vi "Speed Estimation (N Motors).vi"(0 "waveforms":waveform(dbl)[](array[waveform]), 1 "fundamental frequency [Hz]":dbl=50.0, 2 "reset? (F)":bool, 7 "speed estimation settings":cluster{"% overlap":dbl, "algorithm":T2}={"% overlap"=0.0, "algorithm"=enum."3-phase signals"}, 11 "error in (no error)":errorcluster, 12 "nameplate information":T1, 13 "window length (60 s)":dbl=60.0) -> (3 "new data available?":bool, 4 "speed [RPM]":dbl[](array[numeric]), 6 "slip":dbl[](array[numeric]), 15 "error out":errorcluster)   [LabVIEW 2014, in "NI_EP_Motor Monitoring.lvlib"]
doc: "Calculates the motor speed. You must manually select the polymorphic instance you want to use."
uses:
  <vilib>/addons/Electrical Power/Motor Monitoring/NI_EP_Motor Monitoring.lvlib
  <vilib>/addons/Electrical Power/Motor Monitoring/subVIs/ep_Demodulation Algorithm.ctl
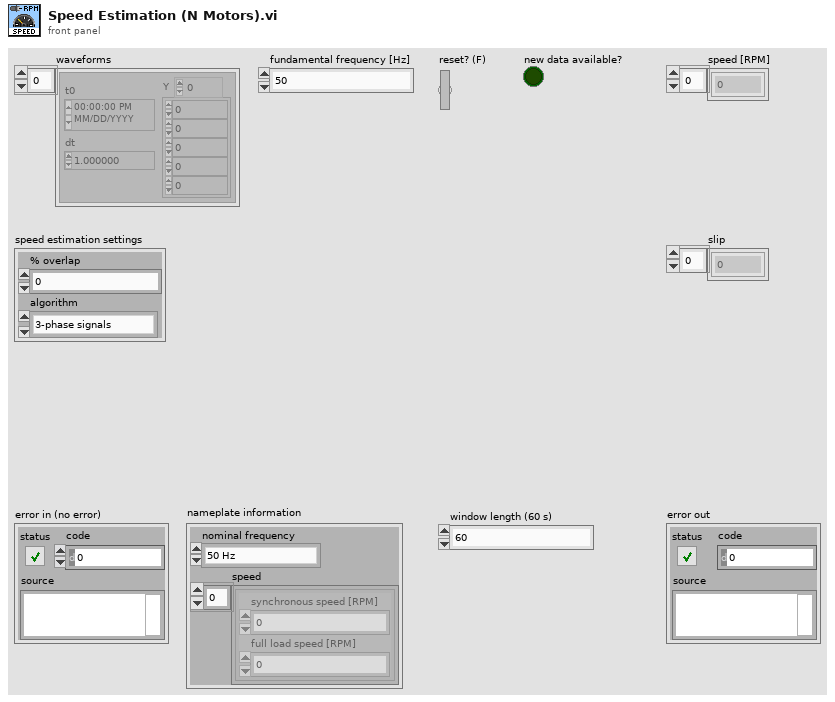
[diagram p1: front panel]
types:
  T1 = cluster{"nominal frequency":enum16{"50 Hz", "60 Hz"}, "speed":cluster{"synchronous speed [RPM]":dbl, "full load speed [RPM]":dbl}[]}
  T2 = typedef "NI_EP_Motor Monitoring.lvlib/ep_Demodulation Algorithm.ctl" = enum16{"1-phase signal", "3-phase signals"}
  T3 = cluster{"block size":i32, "window length [s]":dbl, "dt":dbl}
  T4 = cluster{"synchronous speed [RPM]":dbl, "full load speed [RPM]":dbl}[]
  T5 = typedef "NI_EP_Motor Monitoring.lvlib/ep_Initial Conditions for Speed Estimation.ctl" = cluster{"SVAF state":cluster{"space vector amplitude":dbl, "hilbert state":cluster{"delay conditions":dbl[], "filter conditions":dbl[]}}, "zoom FFT state":cluster{"phase state":dbl, "zoom FFT state":cluster{"zoom settings state":cluster{"zoom":i32, "stop band attenuation":enum16{"84 dB", "96 dB", "120 dB"}, "alias protect in final transition":bool, "oversampling ratio":dbl}, "SML Decimation Filter (complex input) state":cluster{"decimation settings state":cluster{"M":i32, "stop band attenuation":enum16{"84 dB", "96 dB", "120 dB"}, "alias protect in transition band":bool, "oversampling ratio":dbl}, "counter for garbage samples state":i32, "sml_Parameter Setting for Zoom Factor state":cluster{"filter length * interpolation state":i32, "interpolation state":i32, "comb filter order state":i32, "CFIR par state":cluster{"h":dbl[], "M":i32, "N":i32}, "LFIR par state":cluster{"h":dbl[], "M":i32, "N":i32}, "CIC Stages state":i32}, "aal_CIC (complex input) state":cluster{"aal_cascaded moving average (complex input) state":cluster{"states":cdb[], "circular buffers state":cdb[][], "circular buffer counter state":i32}, "aal_moving average with decimation by order (complex input) state":cluster{"residue result state":cdb, "processed data counter state":i32}}, "sml_Cascaded Decimation Filter (complex input) CFIR state":cluster{"unprocessed data state":cdb[], "final conditions state":cdb[][], "sml_M-1 Decimator with IC (complex input) state":cluster{"coefficients in reverse order state":dbl[], "max index for coefficients state":i32}}, "sml_Cascaded Decimation Filter (complex input) LFIR state":cluster{"unprocessed data state":cdb[], "final conditions state":cdb[][], "sml_M-1 Decimator with IC (complex input) state":cluster{"coefficients in reverse order state":dbl[], "max index for coefficients state":i32}}}, "ma_SML Data Packing (complex input) state":cluster{"array getting packed state":cdb[], "last array processed state":cdb[], "index state":i32, "packing parameters state":cluster{i32, "size":i32}}}, "FFT{X} [Vrms]":cdb[]}, "speed state":cluster{"speed [RPM]":dbl, "slip":dbl}, "speed estimation settings":cluster{"% overlap":dbl, "algorithm":T2}, "filter information":cluster{"coefficients":dbl[], "order":i32}, "zoom FFT settings":T6, "last valid window":i32, "fund. frequency for averager":dbl[]}
  T6 = typedef "NI_EP_Motor Monitoring.lvlib/ep_Zoom FFT Settings.ctl" = cluster{"FFT settings":cluster{"window":u16, "Window Size":i32, "FFT Size":i32, "%overlap":dbl}, "zoom settings":cluster{"zoom":i32, "stop band attenuation":enum16{"84 dB", "96 dB", "120 dB"}, "alias protect in final transition":bool, "oversampling ratio":dbl}, "other settings":cluster{"fmod":dbl, "f0":dbl, "df":dbl, "oidx":i32, "olen":i32}, "iterations":i32, "max block size":i32, "fs":dbl}
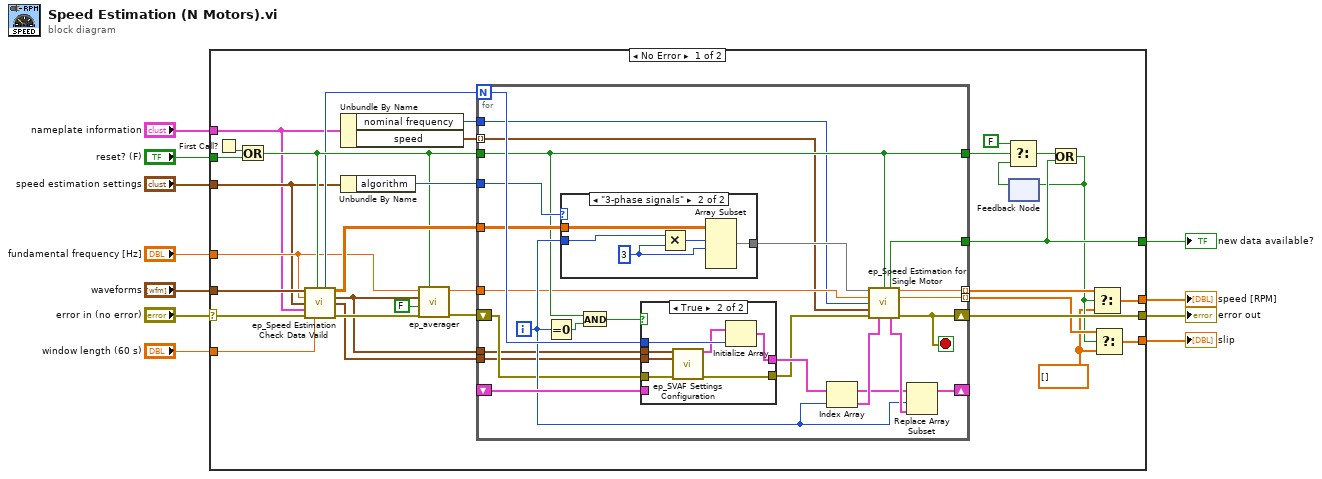
[diagram p0: block diagram]
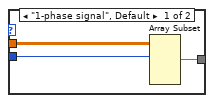
[diagram p3: hidden frame]
diagram:
  n1 = case shown="No Error" "error in (no error)" {
    selector: "error in (no error)" -> [w36 w85]
    tunnel: [w38 w85] -> w10
    tunnel: "fundamental frequency [Hz]" -> [w23 _]
    tunnel: "window length (60 s)" -> [w37 _]
    tunnel: "speed estimation settings" -> [w22 _]
    tunnel: "reset? (F)" -> [w42 _]
    tunnel: "waveforms" -> [w39 _]
    tunnel: "nameplate information" -> [w21 _]
    tunnel: [w26 _] -> w4
    tunnel: [w29 _] -> w2
    tunnel: [w13 _] -> w1
    frame No Error {
      w14 = dbl[] [] ("estimated speed data")
      n2 = First Call?() -> (First Call?: T/F=w43:bool)
      n3 = Or(x=w43, y=w42) -> (x .or. y?=w32:bool)
      n4 = call <vilib>:"ep_Speed Estimation Check Data Vaild.vi"("waveforms"=w39, "reset? (F)"=w32, "fundamental frequency [Hz]"=w23, "speed estimation settings"=w22, "nameplate information"=w21, "error in (no error)"=w36, "window length [s]"=w37) -> ("number of speed"=w24:i32, "signals"=w40:dbl[][], "spectra parameters"=w18:T3, "dup speed estimation settings"=w17:cluster{"% overlap":dbl, "algorithm":T2}, "error out"=w35:errorcluster)  [unwired: 4 in]
      n5 = Unbundle By Name(w21) -> ("nominal frequency"=w20:enum16{"50 Hz", "60 Hz"}, "speed"=w19:T4)
      n6 = Unbundle By Name(w22) -> ("algorithm"=w41:T2)
      n7 = call <vilib>:"ep_averager.vi"("reset? (F)"=w32, "error in (no error)"=w35, "use initial conditions? (F)"=FALSE, "spectra parameters"=w18, "fundamental frequecy"=w23) -> ("error out"=w34:errorcluster, "average"=w33:dbl)  [unwired: 4 in, 1 out]
      n8 = for {
        N: w24 -> [w67]
        shift-right: [w52] -> w38
        shift-left: w34 -> [w51]
        tunnel: w19 -> [w47] mode=indexing
        shift-right: [w63] -> _
        shift-left: _ -> [w64]
        tunnel: w41 -> [w57]
        tunnel: w32 -> [w53]
        tunnel: w40 -> [w59]
        tunnel: w33 -> [w48]
        tunnel: [w54] -> w26
        tunnel: [w56] -> w30 mode=indexing
        tunnel: [w53] -> w25
        tunnel: w18 -> [w49]
        tunnel: w20 -> [w46]
        tunnel: w17 -> [w45]
        tunnel: [w44] -> w16 mode=indexing
        i -> [w55]
        stop <- w52 stop-if-true
        n9 = Equal To 0?(x=w55) -> (x = 0?=w61:bool)
        n10 = case shown="\"3-phase signals\"" w57 {
          tunnel: w55 -> [w78 w83]
          tunnel: w59 -> [w79 w82]
          tunnel: [w77 w80] -> w58
          frame "1-phase signal", Default {
            n11 = Array Subset(array=w79, index (row)=w78) -> (w77:dbl[][])  [unwired: 3 in]
          }
          frame "3-phase signals" {
            w81 = 3 ("y")
            n12 = Multiply(x=w83, y=w81) -> (x*y=w84:i32)
            n13 = Array Subset(array=w82, index (row)=w84, length (row)=w81) -> (w80:dbl[][])  [unwired: 2 in]
          }
        }
        n14 = And(x=w53, y=w61) -> (x .and. y?=w60:bool)
        n15 = case shown="True" w60 {
          tunnel: w67 -> [_ w76]
          tunnel: [w69 w75] -> w62
          tunnel: w64 -> [w69 _]
          tunnel: w51 -> [w68 w73]
          tunnel: [w68 w72] -> w50
          tunnel: w49 -> [_ w71]
          tunnel: w45 -> [_ w70]
          frame False {
          }
          frame True {
            n16 = call <vilib>:"ep_SVAF Settings Configuration.vi"("spectra parameters"=w71, "speed estimation settings"=w70, "error in (no error)"=w73) -> ("initial conditions"=w74:T5, "error out"=w72:errorcluster)  [unwired: 11 in]
            n17 = Initialize Array(w74, w76) -> (w75:T5[])
          }
        }
        n18 = Index Array(array=w62, index=w55) -> (element=w65:T5)
        n19 = call <vilib>:"ep_Speed Estimation for Single Motor.vi"("signals"=w58, "reset? (F)"=w53, "fundamental frequency [Hz]"=w48, "nominal frequency"=w46, "nameplate speed"=w47, "error in (no error)"=w50, "initial conditions"=w65) -> ("new speed available?"=w54:bool, "speed [RPM]"=w56:dbl, "slip"=w44:dbl, "final conditions"=w66:T5, "error out"=w52:errorcluster)  [unwired: 4 in]
        n20 = Replace Array Subset(array=w62, new element=w66, index=w55) -> (w63:T5[])
      }
      n21 = feedback #1() -> (w28:bool)  [unwired: 1 in]
      n22 = Select(t=FALSE, s=w25, f=w28) -> (s? t:f=w27:bool)
      n23 = Or(x=w27, y=w26) -> (x .or. y?=w15:bool)
      n24 = feedback-in #1(w15) -> ()
      n25 = Select(t=w30, s=w15, f=w14) -> (s? t:f=w29:dbl[])
      n26 = Select(t=w16, s=w15, f=w14) -> (s? t:f=w13:dbl[])
    }
    frame Error {
    }
  }
  "error out" <- w10
  "speed [RPM]" <- w2
  "slip" <- w1
  "new data available?" <- w4
